vi "EOL CAN_Template.vi"(7 "Rx Arbitration Id":u32=402522244 format="%.0x", 8 "Error in":errorcluster, 9 "Tx CAN frame":T1={"timestamp"=timestamp(0 s since 1904-01-01), "payload"=[2, 39, 3, 85, 85, 85, 85, 85], "identifier"=402391172, "type"=0, "extended?"=TRUE, "echo?"=FALSE} {"payload" format="%x"; "timestamp" format="%<%.7X\n%x>T"; "type" items=["CAN Data"=0, "CAN Remote"=1, "CAN Bus Error"=2, "CAN 2.0 Data"=8, "CAN FD Data"=16, "CAN FD+BRS Data"=24, "J1939 Data"=192, "Delay"=224, "Log Trigger"=225, "Start Trigger"=226]; "identifier" format="%x"}, 10 "Read Session in":refnum<k21>, 11 "Write Session in":refnum<k21>) -> (0 "Error out":errorcluster, 2 "TxRx Data":string[][](array[string]), 3 "Response Good?":bool)   [LabVIEW 2012]
uses:
  <vilib>/xnet/xnet.llb/XNET Frame Type CAN.ctl
  <vilib>/xnet/xnet.llb/XNET Frame CAN.ctl
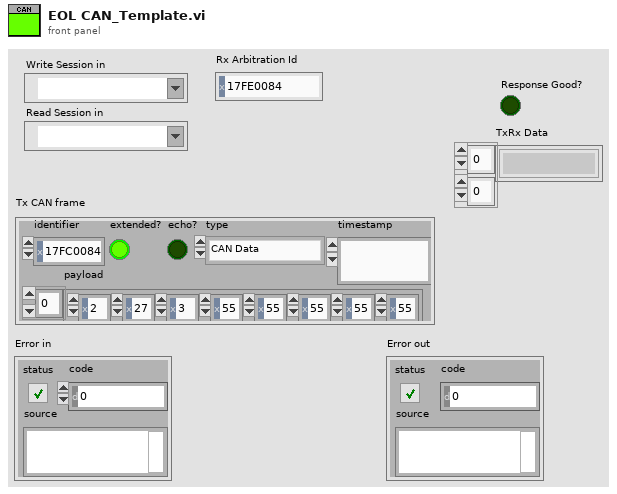
[diagram p1: front panel]
types:
  T1 = typedef "XNET Frame CAN.ctl" = cluster{"timestamp":timestamp, "payload":u8[], "identifier":u32, "type":T2, "extended?":bool, "echo?":bool}
  T2 = typedef "XNET Frame Type CAN.ctl" = u8
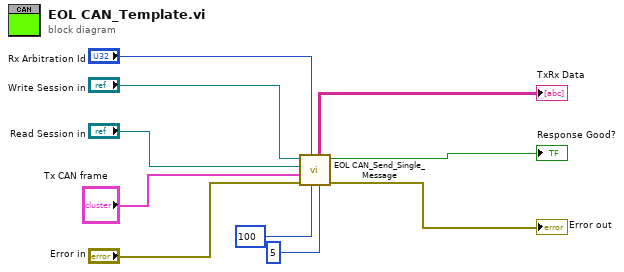
[diagram p0: block diagram]
diagram:
  n1 = call "EOL CAN_Send_Single_Message.vi"("Retries"=5, "Msg Wait Time"=u32 100, "Rx Arbitration Id"="Rx Arbitration Id", "Error in"="Error in", "Tx CAN frame"="Tx CAN frame", "Read Session in"="Read Session in", "Write Session in"="Write Session in") -> ("Error out"=→"Error out":errorcluster, "Response Good?"=→"Response Good?":bool, "TxRx Data"=→"TxRx Data":string[][])  [unwired: 2 out]
